vi "Vision_Right_PC_R3_RIO Test.vi"() -> ()   [LabVIEW 2015]
uses:
  <vilib>/vision/Pattern Matching.llb/IMAQ Curve Parameters.ctl
  <vilib>/vision/Pattern Matching.llb/IMAQ Match Range Setting.ctl
panel:
  in  "INITIAL Search Settings":T3={"Curve Parameters"={"Extraction Mode"=1, "Edge Threshold"=150, "Edge Filter Size"=0, "Min Length"=25, "Row Search Step Size"=15, "Col Search Step Size"=15, "Max Endpoint Gap"=2, "Closed"=TRUE, "Subpixel"=TRUE}, "Match Mode"={"Rotation"=TRUE, "Scale"=TRUE, "Occlusion"=FALSE, "Reserved"=FALSE, "Reserved"=FALSE, "Reserved"=FALSE}, "Range Settings"=[{"Match Constraints"=0, "Min"=-5.0, "Max"=5.0}, {"Match Constraints"=1, "Min"=50.0, "Max"=150.0}, {"Match Constraints"=2, "Min"=0.0, "Max"=0.0}], "Number of Matches"=1, "Minimum Match Score"=900.0, "SubPixel Accuracy"=TRUE, "Adv. Geometric Match Options 2"=[{"Setup Data Item"=20, "Item Value"=0.0}, {"Setup Data Item"=22, "Item Value"=1.0}]} {"Curve Parameters"."Extraction Mode" items=["Normal", "Uniform Regions"]; "Curve Parameters"."Edge Filter Size" items=["Fine", "Normal", "Contour Tracing"]; "Curve Parameters"."Max Endpoint Gap" min=0; "Curve Parameters"."Col Search Step Size" min=1 max=255 step=1; "Curve Parameters"."Row Search Step Size" min=1 max=255 step=1; "Curve Parameters"."Min Length" min=0; "Curve Parameters"."Edge Threshold" min=1 max=350 step=1; "Range Settings"."Max" format="%.2f"; "Range Settings"."Min" format="%.2f"; "Range Settings"."Match Constraints" items=["Rotation Angle (degrees)", "Scale Factor (%)", "Occlusion (%)"]; "Adv. Geometric Match Options 2"."Setup Data Item" items=["Curve Extraction Mode", "Curve Edge Threshold", "Curve Edge Filter Size", "Min Curve Length", "Curve Row Search Step Size", "Curve Col Search Step Size", "Curve Max Endpoint Gap", "Extract Closed Curves", "Enable Subpixel Curve Extraction", "Enable Correlation Score", "Enable Subpixel Accuracy", "Subpixel Iterations", "Subpixel Tolerance", "Initial Match List Length", "Enable Target Template Curve Score", "Min Match Separation Distance", "Min Match Separation Angle", "Min Match Separation Scale", "Max Match Overlap", "Enable Coarse Result", "Enable Calibration Support", "Enable Contrast Reversal", "Search Strategy", "Refinement Match Factor", "Subpixel Match Factor"]}
  in  "Timeout\nfail count":u16=100
  in  "Absolute\nMinimum Scale":dbl=10.0
  in  "Absolute\nMaximum Scale":dbl=300.0
  in  "Absolute\nMinimum Score":dbl=700.0
  in  "ROI_factor(vertical) LR":sgl=3.0
  in  "ROI_factor(Horiztonal) LR":sgl=6.0
  in  "LR to ST\nTransition Scale":sgl=150.0
  in  "SR to LR\nTransition Scale":sgl=70.0
  in  "Score\nCushion":dbl=50.0
  in  "Scale \nCushion":dbl=5.0
  in  "Default SR\nSetting Valuess":T4={"Min Scale"=20.0, "Max Scale"=200.0, "Min Score"=800.0}
  in  "Default LR\nSetting Values":T4={"Min Scale"=50.0, "Max Scale"=200.0, "Min Score"=800.0}
  in  "Default No Lock\nSetting Values":T4={"Min Scale"=20.0, "Max Scale"=250.0, "Min Score"=900.0}
  in  "Main ROI Decay\nper Fail (pixels)":i32=10
  in  "Indivudual Beacon \nCushion (pixels)":sgl=5.0
  out "Valid Scale History":dbl[](array[numeric])=[0.0, 0.0, 60.00346374511719, 0.0, 0.0, 0.0, 0.0, 0.0, 0.0, 0.0, 0.0, 0.0, 0.0, 0.0, 0.0, 0.0, 0.0, 0.0, 0.0, 0.0]
  out "Valid Score History":dbl[](array[numeric])=[0.0, 0.0, 905.1918334960938, 0.0, 0.0, 0.0, 0.0, 0.0, 0.0, 0.0, 0.0, 0.0, 0.0, 0.0, 0.0, 0.0, 0.0, 0.0, 0.0, 0.0]
  out "Valid Match History":bool[](array[boolean])=[FALSE, FALSE, TRUE, FALSE, FALSE, FALSE, FALSE, FALSE, FALSE, FALSE, FALSE, FALSE, FALSE, FALSE, FALSE, FALSE, FALSE, FALSE, FALSE, FALSE]
  out "Current State":u8
  out "Start Up":bool=TRUE
  out "New high Scale":dbl=250.0
  out "New Low Scale":dbl=20.0
  out "New Min Score":dbl=900.0
  out "Current Settings":T3={"Curve Parameters"={"Extraction Mode"=1, "Edge Threshold"=150, "Edge Filter Size"=0, "Min Length"=40, "Row Search Step Size"=15, "Col Search Step Size"=15, "Max Endpoint Gap"=2, "Closed"=TRUE, "Subpixel"=TRUE}, "Match Mode"={"Rotation"=TRUE, "Scale"=TRUE, "Occlusion"=FALSE, "Reserved"=FALSE, "Reserved"=FALSE, "Reserved"=FALSE}, "Range Settings"=[{"Match Constraints"=0, "Min"=-5.0, "Max"=5.0}, {"Match Constraints"=1, "Min"=20.0, "Max"=250.0}, {"Match Constraints"=2, "Min"=0.0, "Max"=0.0}], "Number of Matches"=1, "Minimum Match Score"=900.0, "SubPixel Accuracy"=TRUE, "Adv. Geometric Match Options 2"=[{"Setup Data Item"=20, "Item Value"=0.0}, {"Setup Data Item"=22, "Item Value"=1.0}]} {"Curve Parameters"."Extraction Mode" items=["Normal", "Uniform Regions"]; "Curve Parameters"."Edge Filter Size" items=["Fine", "Normal", "Contour Tracing"]; "Curve Parameters"."Max Endpoint Gap" min=0; "Curve Parameters"."Col Search Step Size" min=1 max=255 step=1; "Curve Parameters"."Row Search Step Size" min=1 max=255 step=1; "Curve Parameters"."Min Length" min=0; "Curve Parameters"."Edge Threshold" min=1 max=350 step=1; "Range Settings"."Max" format="%.2f"; "Range Settings"."Min" format="%.2f"; "Range Settings"."Match Constraints" items=["Rotation Angle (degrees)", "Scale Factor (%)", "Occlusion (%)"]}
  out "Current Score":sgl
  out "Current Scale":sgl
  out "Avg Scale":dbl=100.0
  out "Avg Score":dbl=750.0
  out "next ROI Rectangle 2":cluster{dbl, dbl, dbl, dbl, dbl}={87.0, 139.0, 527.0, 319.0, 0.0}
  in  "ROI_factor(vertical) SR":sgl=1.2
  in  "ROI_factor(Horiztonal) SR":sgl=6.0
  in  "Valid Treshold\nfor Lock":i16=5
  in  "History Size":i32=20
  out "Lock Status":bool
  out "SR Found":bool
  out "LR Found":bool
  out "Beacon 4 Data":cluster{"X":sgl, "Y":sgl}
  out "Beacon 3 Data":cluster{"X":sgl, "Y":sgl}={"X"=404.75333, "Y"=236.50656}
  out "Beacon 2 Data":cluster{"X":sgl, "Y":sgl}={"X"=305.31543, "Y"=230.27802}
  out "Beacon 1 Data":cluster{"X":sgl, "Y":sgl}={"X"=212.05559, "Y"=225.89603}
  out "Beacon 0 Data":cluster{"X":sgl, "Y":sgl}={"X"=128.98677, "Y"=232.05302}
  out "dT":u32=499
  out "Left Beacon Bools":bool[](array[boolean])
  out "Y Values":sgl[](array[numeric])=[232.05302, 225.89603, 230.27802, 236.50656, 0.0]
  out "X Values":sgl[](array[numeric])=[128.98677, 212.05559, 305.31543, 404.75333, 0.0]
  # "CURRENT VALUES"
  # "ADAPTIVE SETTINGS"
  # "Range"
  # "Range"
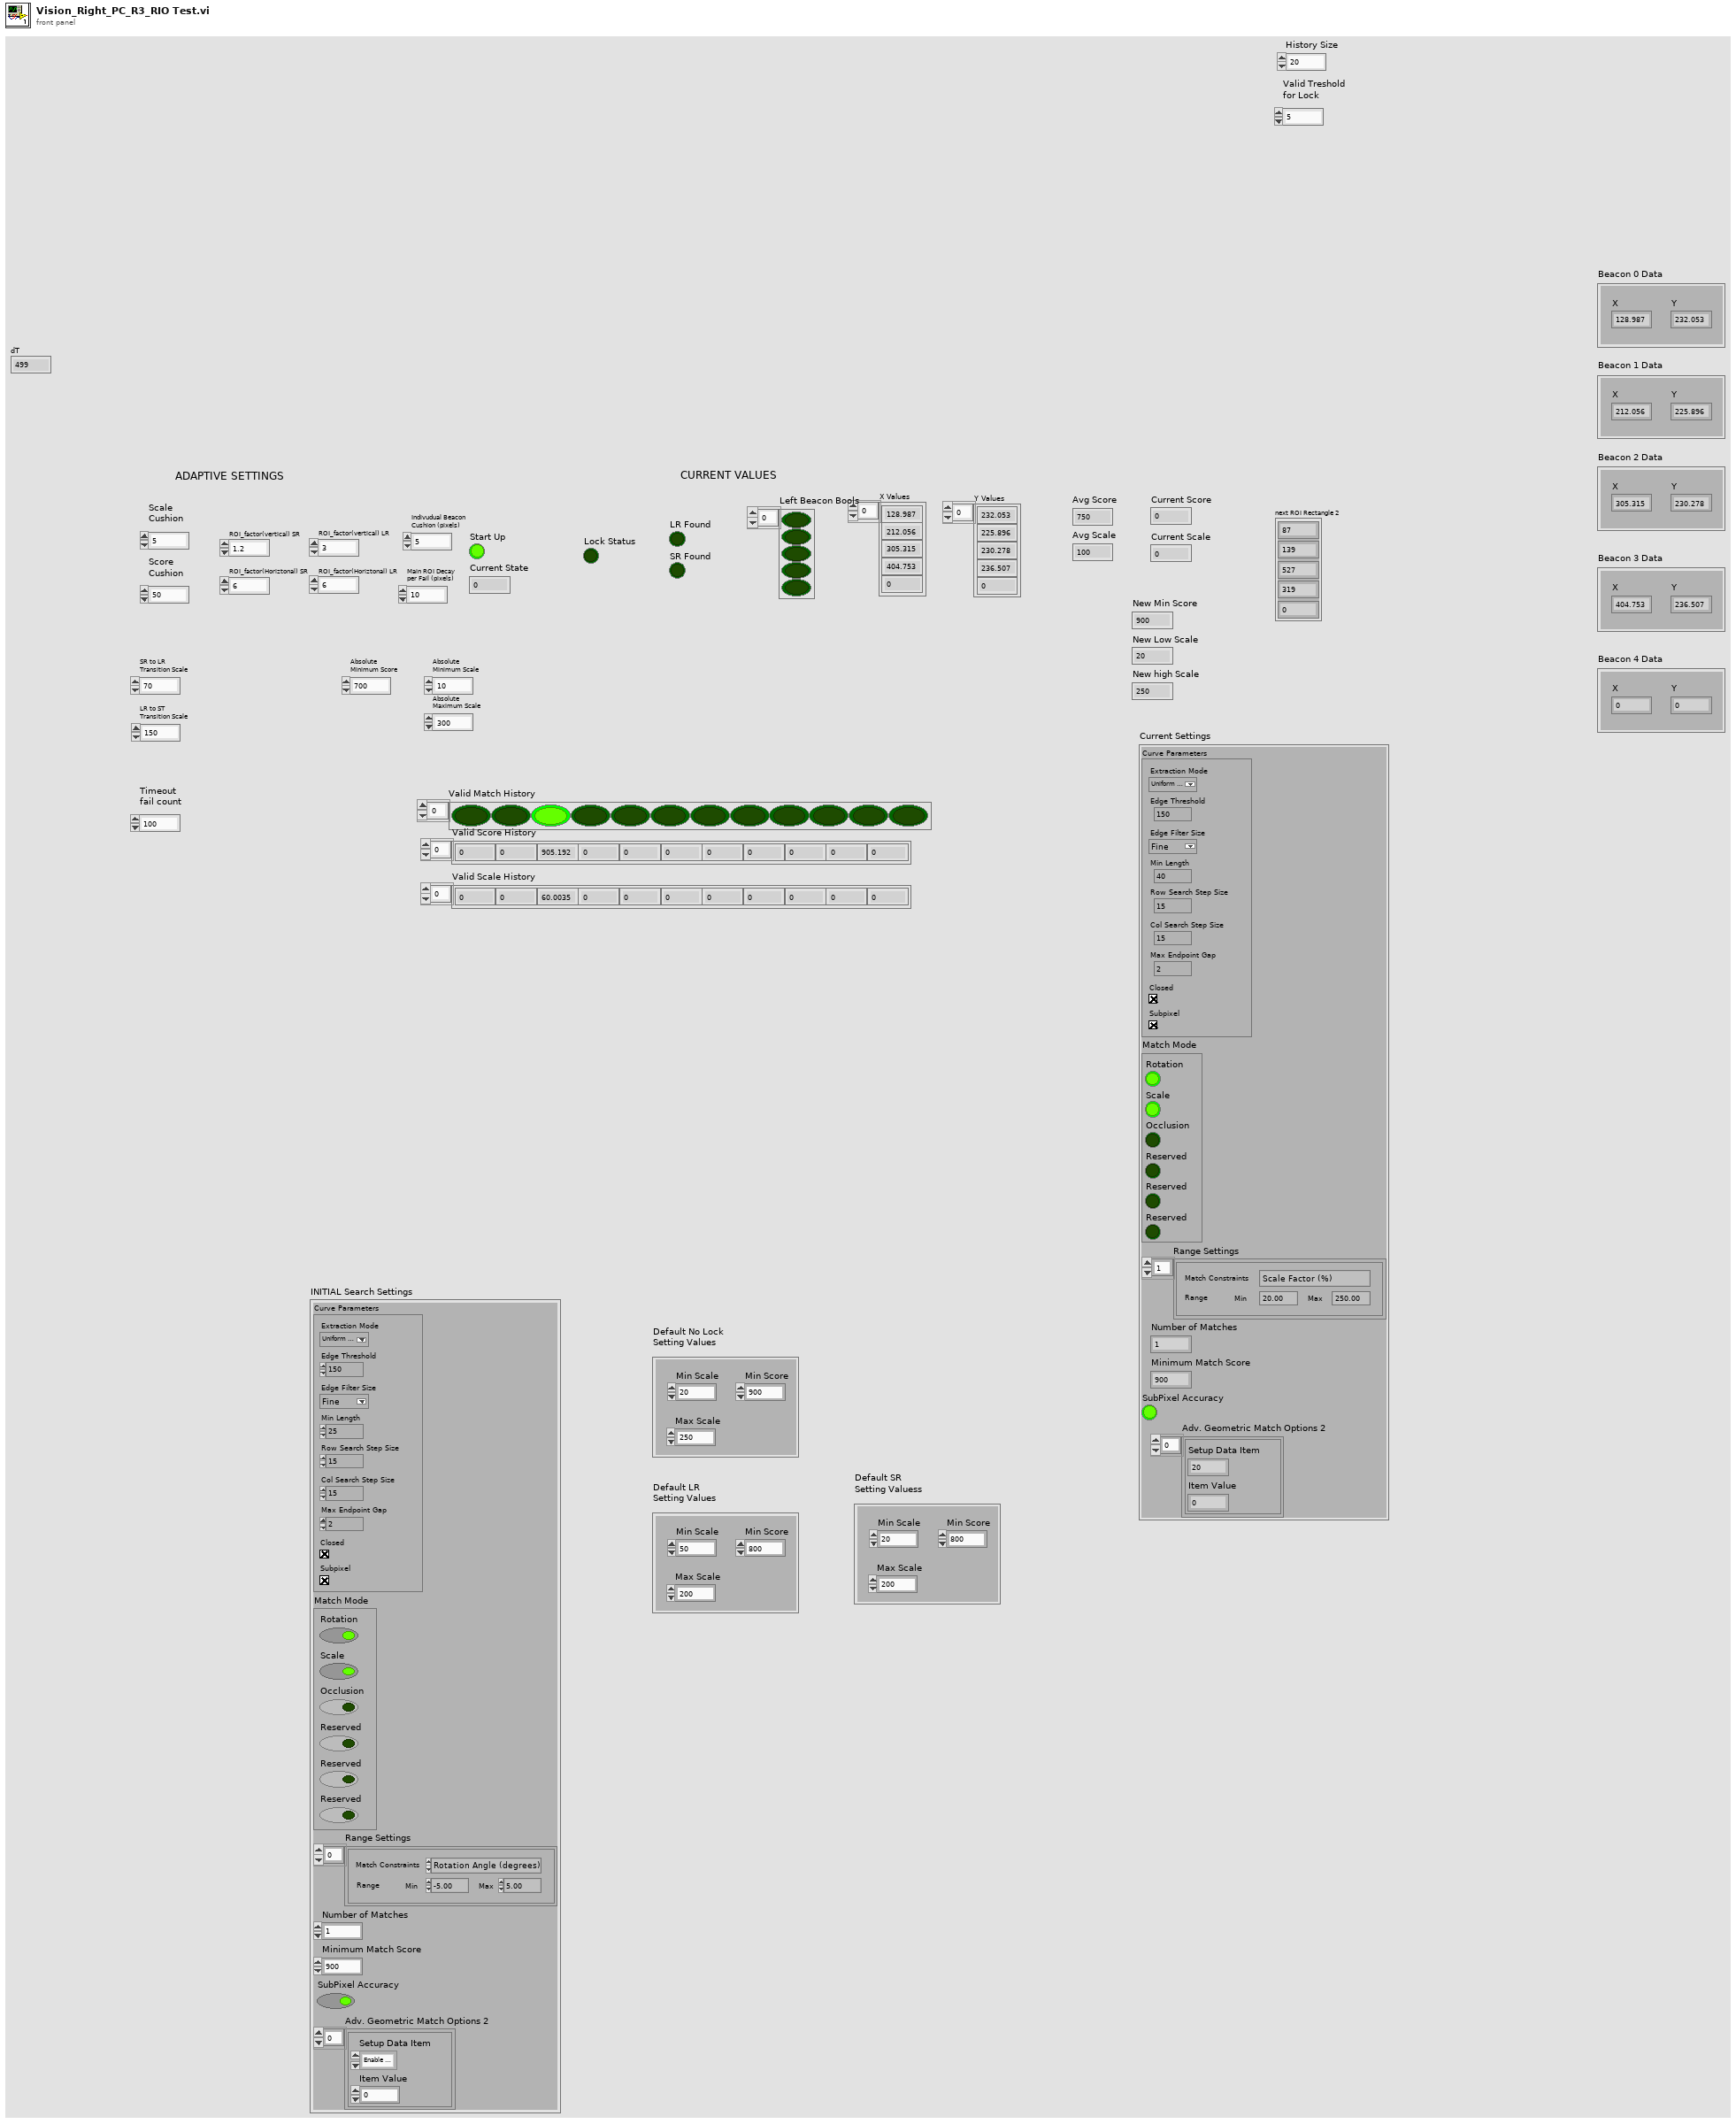
[diagram p1: front panel]
types:
  T1 = typedef "IMAQ Curve Parameters.ctl" = cluster{"Extraction Mode":u32, "Edge Threshold":i32, "Edge Filter Size":u32, "Min Length":i32, "Row Search Step Size":i32, "Col Search Step Size":i32, "Max Endpoint Gap":i32, "Closed":bool, "Subpixel":bool}
  T2 = typedef "IMAQ Match Range Setting.ctl" = cluster{"Match Constraints":u32, "Min":dbl, "Max":dbl}
  T3 = cluster{"Curve Parameters":T1, "Match Mode":cluster{"Rotation":bool, "Scale":bool, "Occlusion":bool, "Reserved":bool, "Reserved":bool, "Reserved":bool}, "Range Settings":T2[], "Number of Matches":i32, "Minimum Match Score":sgl, "SubPixel Accuracy":bool, "Adv. Geometric Match Options 2":cluster{"Setup Data Item":u16, "Item Value":dbl}[]}
  T4 = cluster{"Min Scale":dbl, "Max Scale":dbl, "Min Score":dbl}
  T5 = typedef "Image Type" = u32
  T6 = typedef "ROI Descriptor" = cluster{"Global Rectangle":i32[], "Contours":cluster{"ID":enum32{"External", "Internal"}, "Type":u32, "Coordinates":i32[]}[]}
  T7 = typedef "IMAQ Image.ctl" = refnum<image>
  T8 = typedef "IMAQ GM Match Report.ctl" = cluster{"Position":cluster{"x":sgl, "y":sgl}, "Angle":sgl, "Scale":sgl, "Score":sgl, "Bounding Box":cluster{"x":sgl, "y":sgl}[], "Contrast Reversed":bool, "Occlusion %":sgl, "Template Target Curve Score":sgl, "Target Template Curve Score":sgl, "Correlation Score":sgl}
  T9 = cluster{"Matches (Geometric Matching 1)[0]":T8, "Matches (Geometric Matching 1)[1]":T8, "Matches (Geometric Matching 1)[2]":T8, "Matches (Geometric Matching 1)[3]":T8, "Matches (Geometric Matching 1)[4]":T8, "Matches (Geometric Matching 1)[5]":T8, "Matches (Geometric Matching 1)[6]":T8, "Matches (Geometric Matching 1)[7]":T8, "Matches (Geometric Matching 1)[8]":T8}
  T10 = cluster{"Bounding Box[0]":cluster{"x":sgl, "y":sgl}, "Bounding Box[1]":cluster{"x":sgl, "y":sgl}, "Bounding Box[2]":cluster{"x":sgl, "y":sgl}, "Bounding Box[3]":cluster{"x":sgl, "y":sgl}, "Bounding Box[4]":cluster{"x":sgl, "y":sgl}, "Bounding Box[5]":cluster{"x":sgl, "y":sgl}, "Bounding Box[6]":cluster{"x":sgl, "y":sgl}, "Bounding Box[7]":cluster{"x":sgl, "y":sgl}, "Bounding Box[8]":cluster{"x":sgl, "y":sgl}}
  T11 = typedef "IMAQ Rectangle" = cluster{"Left":i32, "Top":i32, "Right":i32, "Bottom":i32, "Rotation":dbl}
  T12 = cluster{"index":u32, "Min Scale":dbl, "Max Scale":dbl}
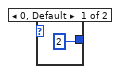
[diagram p2: hidden frame]
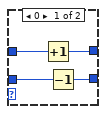
[diagram p4: hidden frame]
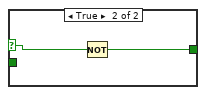
[diagram p5: hidden frame]
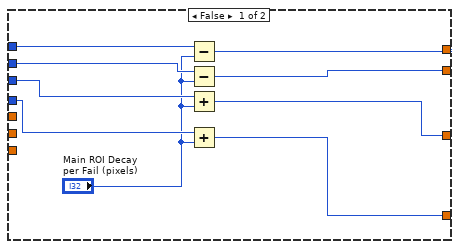
[diagram p6: hidden frame]
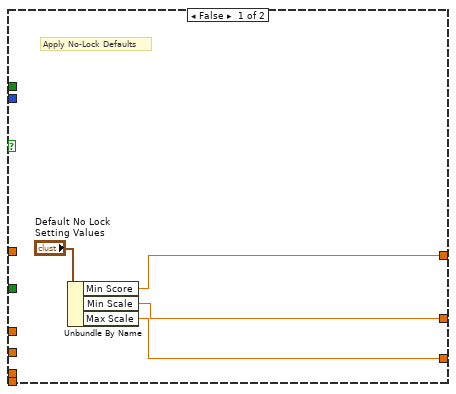
[diagram p11: hidden frame]
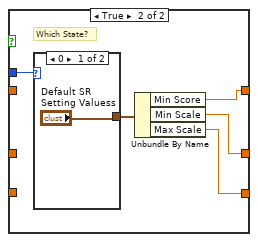
[diagram p12: hidden frame]
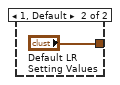
[diagram p13: hidden frame]
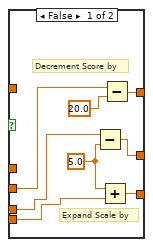
[diagram p14: hidden frame]
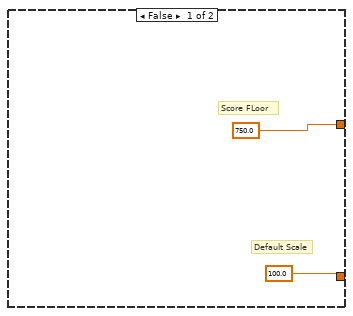
[diagram p15: hidden frame]
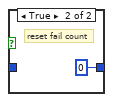
[diagram p17: hidden frame]
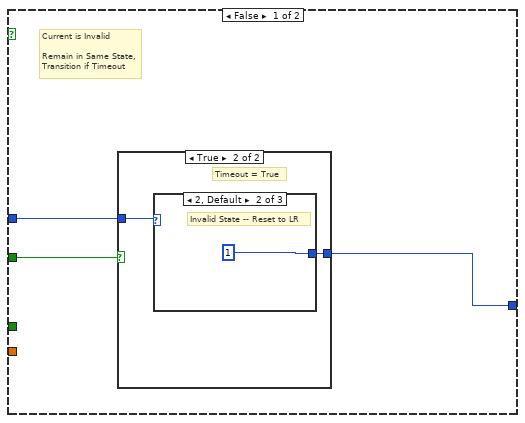
[diagram p18: hidden frame]
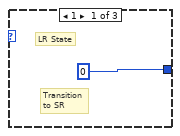
[diagram p20: hidden frame]
diagram:
  # "0 = Close Range (3)\n1 = Regular (5)"
  n1 = flat-sequence {
    tunnel: [w32] -> w12
    tunnel: [w29] -> w11
    tunnel: [w28] -> w10
    tunnel: ["INITIAL Search Settings"] -> w9
    tunnel: [u8 0] -> w8
    tunnel: [w24] -> w7
    tunnel: [FALSE] -> w6
    tunnel: [TRUE] -> w5
    tunnel: [w20] -> w4
    tunnel: [u16 0] -> w3
    tunnel: [w15] -> w2
    tunnel: [w14] -> w1
    tunnel: w12 -> [w46]
    tunnel: w11 -> [w51]
    tunnel: w10 -> [w49]
    tunnel: w9 -> [w47]
    tunnel: w8 -> [w50]
    tunnel: w7 -> [w48]
    tunnel: w6 -> [w45]
    tunnel: w5 -> [w44]
    tunnel: w4 -> [w43]
    tunnel: w3 -> [w42]
    tunnel: w2 -> [w41]
    tunnel: w1 -> [w40]
    frame #0 {
      w31 = T5 0 items=["Grayscale (U8)", "Grayscale (I16)", "Grayscale (SGL)", "Complex (CSG)", "RGB (U32)", "HSL (U32)", "RGB (U64)", "Grayscale (U16)"] ("Image Type")
      # "Score History"
      # "Scale History"
      # "Fail Counter"
      # "Valid Match History\n(main beacon)"
      # "Lock Status"
      # "Sub Beacon Search Array"
      # "Template State"
      # "Search Parameters"
      # "StartUp = True"
      # "Initial ROI Descriptor"
      # "INITIALIZE"
      n2 = Bundle(0, 0, 640, 480, 0) -> (w33:cluster{i32, i32, i32, i32, i32})  [unwired: 1 in]
      n3 = call "IMAQ Convert Rectangle to ROI"("Rectangle"=w33) -> ("ROI Descriptor"=w32:T6)  [unwired: 8 in, 1 out]
      n4 = Initialize Array(FALSE, 5 ("dimension size")) -> (w24:bool[])
      n5 = Initialize Array(FALSE, "History Size") -> (w20:bool[])
      n6 = Initialize Array(0.0, "History Size") -> (w14:dbl[])
      n7 = Initialize Array(0.0, "History Size") -> (w15:dbl[])
      n8 = call "IMAQ Create"("Image Name"="Right_Image", "Image Type"=w31) -> ("New Image"=w28:T7, "error out"=w29:errorcluster)  [unwired: 3 in]
    }
    frame #1 {
      # "Fail Counter"
      # "Template State"
      # "Score History"
      # "Scale History"
      # "Valid Match History\n(main beacon)"
      # "Lock Status"
      # "Sub Beacon Search Array"
      # "StartUp"
      n9 = call "Tick Count3"() -> ("Tick Count(uSec)"=w39:u32)
      n10 = while {
        tunnel: w51 -> [w84]
        shift-right: [w76] -> _
        shift-left: w50 -> [w80]
        shift-right: [w68] -> _
        shift-left: w44 -> [w69]
        tunnel: w49 -> [w81]
        shift-right: [w67] -> _
        shift-left: w48 -> [w79]
        shift-right: [w72] -> _
        shift-left: w47 -> [w73]
        shift-right: [w70] -> _
        shift-left: w46 -> [w71]
        shift-right: [w66] -> _
        shift-left: w45 -> [_]
        shift-right: [w63] -> _
        shift-left: w43 -> [w78]
        shift-right: [w62] -> _
        shift-left: w42 -> [w77]
        shift-right: [w64] -> _
        shift-left: w41 -> [w75]
        shift-right: [w65] -> _
        shift-left: w40 -> [w74]
        shift-right: [w59] -> _
        shift-left: w39 -> [w60]
        stop <- FALSE stop-if-true
        n11 = flat-sequence {
          tunnel: w84 -> [w88]
          tunnel: [w87] -> w83
          tunnel: [w86] -> w82
          tunnel: [w85] -> w52
          tunnel: w83 -> [w271]
          tunnel: w82 -> [w270]
          tunnel: w81 -> [w254]
          tunnel: w69 -> [w269]
          tunnel: w80 -> [w127]
          tunnel: w79 -> [w268]
          tunnel: w73 -> [w126]
          tunnel: w71 -> [w267]
          tunnel: w78 -> [w208]
          tunnel: w73 -> [w188]
          tunnel: w77 -> [w204]
          tunnel: [w114] -> w76
          tunnel: w75 -> [w139]
          tunnel: w74 -> [w140]
          tunnel: [w186] -> w72
          tunnel: w71 -> [w159]
          tunnel: w69 -> [w152]
          tunnel: [w149] -> w65
          tunnel: [w148] -> w64
          tunnel: [w147] -> w63
          tunnel: [w146] -> w62
          tunnel: w60 -> [w142]
          tunnel: [w157] -> w58
          tunnel: [w156] -> w57
          tunnel: [w151] -> w56
          tunnel: [w150] -> w55
          tunnel: [w118] -> w54
          tunnel: [w141] -> w53
          tunnel: w52 -> [w91]
          tunnel: [w701] -> w59
          tunnel: [w702] -> w66
          tunnel: [w703] -> w67
          tunnel: [w704] -> w68
          tunnel: [w705] -> _
          tunnel: [w706] -> w70
          tunnel: w58 -> [w706]
          tunnel: w57 -> [w705]
          tunnel: w56 -> [w704]
          tunnel: w55 -> [w703]
          tunnel: w54 -> [w702]
          tunnel: w53 -> [w701]
          frame #0 {
            # "Take Image"
            n12 = shared-variable "RT myRIO Target - Overlord\\Localization_Variables_r0.lvlib\\Right Servo Angle_Current"() -> (w85:dbl)  [unwired: 1 in, 1 out]
            n13 = call "Right Camera Acquisition"("error in"=w88) -> ("Image Out"=w86:T7, "error out"=w87:errorcluster)  [unwired: 24 in, 1 out]
          }
          frame #1 {
            w89 = sgl 240.0 ("y")
            w90 = sgl 320.0 ("y")
            w189 = u32 1 ("index")
            (unwired) 0
            # "Apply Limits to Settings"
            # "Choose ROI Scale Factor"
            # "Current Min\n& Max Scale"
            # "fail count out"
            # "Next State"
            # "Have fail count threshold to reset to worst case scenario settings, have treshold less than timeout"
            # "False case*********"
            # "Make new templates for sub beacons based on \noriginal template... import pic to express VI\n\n\nUse scale window for smaller beacons"
            # "Outer Beacon\nIndexes"
            # "Build ROI for Individual Beacons Based on Main Bounding Box"
            # "Maybe check for main here"
            # "Startup FLag"
            # "Pull Down Startup IF Already True and Lock\nOtherwise don't update"
            # "ROI"
            # "State Change"
            # "Next Settings"
            # "Settings out"
            # "Scale"
            # "Min Score"
            # "Lower Scale"
            # "Upper Scale"
            # "If Locked"
            # "Average Scale"
            # "Average Score"
            # "Only Calculate\nAvg if 2 available"
            # "Valid  Ccount\n(up to 3)"
            # "Only Calculate MOving Avg\nif xx% of previous positions were valid"
            # "Update Avg Score & Scale"
            # "Timeout"
            # "Update Fail Counter"
            # "Next State"
            # "Settings"
            # "Update Template State"
            # "Update Main ROI"
            # "Update Search Setting Values"
            # "Current Match is Valid \nIF: \n     Main Found\n     At Least 2 or 3 beacons"
            # "****# of previous in history that must be true\nin order for position to be considered \"locked\""
            # "Shift & Insert Current Valid Match"
            # "Update Lock Status & Shift Arrays"
            # "Main Found"
            # "Update Beacon Outputs"
            # "Valid Match"
            # "Valid Match"
            # "Valid Match"
            # "Valid Match"
            # "Assume 0 Angle"
            # "Starting X Lower Bound"
            # "Length of\nIndividual Beacon ROI"
            # "Length of Bounding Box"
            # "LR Found"
            # "SR Found"
            # "Valid Match"
            # "Only Attempt Sub If Supposed To"
            # "Search for Sub Beacons"
            # "Force SR if Start Up"
            # "Choose Template (SR or LR)\n& Search"
            n14 = case shown="True" w269 {
              tunnel: w127 -> [w635 _]
              tunnel: [w635 u8 1] -> w95
              frame False {
                # "Not Start Up\n\nDon't Update \nTemplate State"
              }
              frame True {
                # "Start Up --> SR"
              }
            }
            "Current State" <- w95
            n15 = shared-variable "RT myRIO Target - Overlord\\Localization_Variables_r0.lvlib\\Right Servo Angle_Image"(w91) -> ()  [unwired: 1 in, 1 out]
            n16 = case shown="1" w95 {
              tunnel: w271 -> [w651 w683]
              tunnel: w270 -> [w650 w682]
              tunnel: w254 -> [w649 w681]
              tunnel: w268 -> [w646 w677]
              tunnel: w126 -> [w645 w671]
              tunnel: w267 -> [w644 w670]
              tunnel: [w643 w676] -> w150
              tunnel: [sgl 3.0 ("y") sgl 5.0 ("y")] -> w253
              tunnel: [w641 w673] -> w155
              tunnel: [w640 w672] -> w158
              tunnel: [w639 FALSE] -> w216
              tunnel: [FALSE w675] -> w217
              frame 0, Default {
                # "Sub-Beacon Search\nArray"
                n17 = call "Left Camera - Short Range"("Image In"=w650, "Image Dst"=w649, "ROI Descriptor (Geometric Matching 1)"=w644, "Settings (Geometric Matching 1)"=w645, "Template File Path (Geometric Matching 1)"=path "/home/lvuser/natinst/bin/BeaconTemplates_TEST/Close Range (3 subs).png", "error in"=w651) -> ("Image Out"=w641:T7, "Matches (Geometric Matching 1)"=w640:T8[], "Number of Matches (Geometric Matching 1)"=w648:i32)  [unwired: 18 in, 1 out]
                n18 = Equal?(x=w648, y=1) -> (x = y?=w639:bool)
                n19 = case shown="True" w639 {
                  tunnel: w646 -> [w659 w663]
                  tunnel: [w652 w660] -> w643
                  frame False {
                    w653 = FALSE
                    # "No Main Found,\nDon't Search any Subs"
                    n20 = Replace Array Subset(array=w659, new element #1=w653, index #1=0 ("y"), new element #2=w653, index #2=1 ("y"), new element #3=w653, index #3=2 ("y"), new element #4=w653, index #4=3 ("y"), new element #5=w653, index #5=4 ("y")) -> (w652:bool[])
                  }
                  frame True {
                    w661 = TRUE
                    w662 = FALSE
                    # "Search for Middle 3 Subs"
                    n21 = Replace Array Subset(array=w663, new element #1=w662, index #1=0 ("y"), new element #2=w661, index #2=1 ("y"), new element #3=w661, index #3=2 ("y"), new element #4=w661, index #4=3 ("y"), new element #5=w662, index #5=4 ("y")) -> (w660:bool[])
                  }
                }
              }
              frame 1 {
                # "Main (5) Pattern"
                n22 = call "Left Camera - Long Range"("Image In"=w682, "Image Dst"=w681, "ROI Descriptor (Geometric Matching 1)"=w670, "Settings (Geometric Matching 1)"=w671, "Template File Path (Geometric Matching 1)"=path "/home/lvuser/natinst/bin/BeaconTemplates_TEST/Main Beacon_8ft - 320_240.png", "error in"=w683) -> ("Image Out"=w673:T7, "Matches (Geometric Matching 1)"=w672:T8[], "Number of Matches (Geometric Matching 1)"=w678:i32)  [unwired: 18 in, 1 out]
                n23 = Equal?(x=w678, y=1) -> (x = y?=w675:bool)
                n24 = case shown="True" w675 {
                  tunnel: w677 -> [w691 w693]
                  tunnel: [w684 w692] -> w676
                  frame False {
                    w685 = FALSE
                    # "F"
                    # "No Main Found,\nDon't Search any Subs"
                    n25 = Replace Array Subset(array=w691, new element #1=w685, index #1=0 ("y"), new element #2=w685, index #2=1 ("y"), new element #3=w685, index #3=2 ("y"), new element #4=w685, index #4=3 ("y"), new element #5=w685, index #5=4 ("y")) -> (w684:bool[])
                  }
                  frame True {
                    w694 = TRUE
                    # "T"
                    # "Search for ALL Beacons"
                    n26 = Replace Array Subset(array=w693, new element #1=w694, index #1=0 ("y"), new element #2=w694, index #2=1 ("y"), new element #3=w694, index #3=2 ("y"), new element #4=w694, index #4=3 ("y"), new element #5=w694, index #5=4 ("y")) -> (w692:bool[])
                  }
                }
              }
            }
            "LR Found" <- w217
            "SR Found" <- w216
            n27 = Array To Cluster(array=w158) -> (cluster=w138:T9)
            n28 = Unbundle By Name(w138) -> ("Matches (Geometric Matching 1)[0].Bounding Box"=w255:cluster{"x":sgl, "y":sgl}[], "Matches (Geometric Matching 1)[0].Scale"=w195:sgl, "Matches (Geometric Matching 1)[0].Correlation Score"=w154:sgl)
            "Current Scale" <- w195
            "Current Score" <- w154
            n29 = Or(x=w217, y=w216) -> (x .or. y?=w209:bool)
            n30 = Array To Cluster(array=w255) -> (cluster=w266:T10)
            n31 = Unbundle By Name(w266) -> ("Bounding Box[0].x"=w250:sgl, "Bounding Box[0].y"=w137:sgl, "Bounding Box[2].x"=w248:sgl, "Bounding Box[2].y"=w135:sgl)
            n32 = Subtract(x=w248, y=w250) -> (x-y=w252:sgl)
            n33 = case shown="1, Default" w95 {
              tunnel: [w279 w283] -> w130
              tunnel: [w278 w282] -> w129
              tunnel: 0 -> [w281 w283]
              tunnel: 4 -> [w280 w282]
              frame 0 {
                n34 = Increment(x=w281) -> (x+1=w279:i32)
                n35 = Decrement(x=w280) -> (x-1=w278:i32)
              }
              frame 1, Default {
              }
            }
            n36 = Divide(x=w252, y=w253) -> (x/y=w249:sgl)
            n37 = Subtract(x=w137, y="Indivudual Beacon \nCushion (pixels)") -> (x-y=w136:sgl)
            n38 = Add(x="Indivudual Beacon \nCushion (pixels)", y=w135) -> (x+y=w134:sgl)
            n39 = for {
              N: 5 -> [_]
              tunnel: w150 -> [w496] mode=indexing
              shift-right: [w480] -> _
              shift-left: w250 -> [w495]
              tunnel: w249 -> [w494]
              tunnel: w136 -> [w493]
              tunnel: w134 -> [w492]
              tunnel: [w489] -> w131 mode=indexing
              tunnel: w130 -> [w486]
              tunnel: w129 -> [w487]
              tunnel: "Indivudual Beacon \nCushion (pixels)" -> [w477]
              i -> [w488]
              # "Apply Horizontal Cushion to Outer Beacons"
              # "Divide Bounding Box"
              # "Upper Bound of Current is\nLower Bound for Next"
              # "Build ROI\nDescriptor"
              n40 = case shown="True" w496 {
                tunnel: w495 -> [w509 w510]
                tunnel: w494 -> [_ w512]
                tunnel: [w509 w511] -> w478
                tunnel: [w509 w510] -> w483
                frame False {
                  # "Don't Care"
                }
                frame True {
                  # "X Lower Bound"
                  n41 = Add(x=w510, y=w512) -> (x+y=w511:sgl)
                }
              }
              n42 = Equal?(x=w488, y=w486) -> (x = y?=w485:bool)
              n43 = case shown="True" w485 {
                tunnel: w483 -> [w504 w508]
                tunnel: [w504 w505] -> w482
                tunnel: [w503 w506] -> w479
                tunnel: w478 -> [w503 w506]
                tunnel: w477 -> [_ w507]
                frame False {
                }
                frame True {
                  n44 = Subtract(x=w508, y=w507) -> (x-y=w505:sgl)
                }
              }
              n45 = Equal?(x=w488, y=w487) -> (x = y?=w484:bool)
              n46 = case shown="True" w484 {
                tunnel: w482 -> [w498 w502]
                tunnel: [w498 w501] -> w481
                tunnel: [w497 w499] -> w480
                tunnel: w479 -> [w497 w499]
                tunnel: w477 -> [_ w500]
                frame False {
                }
                frame True {
                  n47 = Add(x=w502, y=w500) -> (x+y=w501:sgl)
                }
              }
              n48 = Bundle("x"=w481, w493, "x"=w480, w492, 0) -> (w490:cluster{"x":sgl, sgl, "x":sgl, sgl, i32})  [unwired: 1 in]
              n49 = call "IMAQ Convert Rectangle to ROI"("Rectangle"=w490) -> ("ROI Descriptor"=w489:T6)  [unwired: 8 in, 1 out]
            }
            n50 = Index Array(array=w150, index=1) -> (element=w259:bool)
            n51 = Index Array(array=w131, index=1) -> (element=w241:T6)
            n52 = Index Array(array=w150, index=2) -> (element=w258:bool)
            n53 = Index Array(array=w131, index=2) -> (element=w240:T6)
            n54 = Index Array(array=w150, index=0) -> (element=w265:bool)
            n55 = Index Array(array=w131, index=3) -> (element=w239:T6)
            n56 = Index Array(array=w150, index=3) -> (element=w257:bool)
            n57 = Index Array(array=w131, index=4) -> (element=w238:T6)
            n58 = Index Array(array=w131, index=0) -> (element=w242:T6)
            n59 = Index Array(array=w150, index=4) -> (element=w256:bool)
            n60 = case shown="True" w259 {
              tunnel: w241 -> [_ w601]
              tunnel: w155 -> [_ w600]
              tunnel: w254 -> [_ w599]
              tunnel: [FALSE w592] -> w236
              tunnel: w95 -> [_ w591]
              tunnel: w126 -> [_ w590]
              frame False {
              }
              frame True {
                # "Update Beacon Coordinates if Found"
                n61 = case shown="1, Default" w591 {
                  tunnel: w601 -> [w606 w615]
                  tunnel: w600 -> [w608 w614]
                  tunnel: w599 -> [w607 w613]
                  tunnel: [w604 w612] -> w594
                  tunnel: [w605 w611] -> w593
                  tunnel: w590 -> [w603 w610]
                  frame 0 {
                    n62 = call "Mid Left Match Short Range"("Image In"=w608, "Image Dst"=w607, "ROI Descriptor (Geometric Matching 1)"=w606, "Settings (Geometric Matching 1)"=w603, "Template File Path (Geometric Matching 1)"=path "/home/lvuser/natinst/bin/BeaconTemplates_TEST/sub2_SR.png") -> ("Matches (Geometric Matching 1)"=w605:T8[], "Number of Matches (Geometric Matching 1)"=w604:i32)  [unwired: 19 in, 2 out]
                  }
                  frame 1, Default {
                    n63 = call "Mid Left Match Long Range"("Image In"=w614, "Image Dst"=w613, "ROI Descriptor (Geometric Matching 1)"=w615, "Settings (Geometric Matching 1)"=w610, "Template File Path (Geometric Matching 1)"=path "/home/lvuser/natinst/bin/BeaconTemplates_TEST/sub2_8ft - 320_240.png") -> ("Matches (Geometric Matching 1)"=w611:T8[], "Number of Matches (Geometric Matching 1)"=w612:i32)  [unwired: 19 in, 2 out]
                  }
                }
                n64 = Array To Cluster(array=w593) -> (cluster=w598:T9)
                n65 = Equal?(x=w594, y=1) -> (x = y?=w592:bool)
                n66 = Unbundle By Name(w598) -> ("Matches (Geometric Matching 1)[0].Position.x"=w596:sgl, "Matches (Geometric Matching 1)[0].Position.y"=w595:sgl)
                n67 = case shown="True" w592 {
                  tunnel: w596 -> [_ w618]
                  tunnel: w595 -> [_ w617]
                  frame False {
                  }
                  frame True {
                    n68 = Bundle("x"=w618, "y"=w617) -> (→"Beacon 1 Data":cluster{"x":sgl, "y":sgl})  [unwired: 1 in]
                  }
                }
              }
            }
            n69 = case shown="True" w258 {
              tunnel: w240 -> [_ w562]
              tunnel: w155 -> [_ w571]
              tunnel: w254 -> [_ w570]
              tunnel: [FALSE w563] -> w235
              tunnel: w95 -> [_ w561]
              tunnel: w126 -> [_ w560]
              frame False {
              }
              frame True {
                # "Update Beacon Coordinates if Found"
                n70 = case shown="1, Default" w561 {
                  tunnel: w571 -> [w578 w585]
                  tunnel: w570 -> [w577 w584]
                  tunnel: [w575 w583] -> w565
                  tunnel: [w574 w582] -> w564
                  tunnel: w562 -> [w576 w581]
                  tunnel: w560 -> [w573 w580]
                  frame 0 {
                    n71 = call "Middle Match Short Range"("Image In"=w578, "Image Dst"=w577, "ROI Descriptor (Geometric Matching 1)"=w576, "Settings (Geometric Matching 1)"=w573, "Template File Path (Geometric Matching 1)"=path "/home/lvuser/natinst/bin/BeaconTemplates_TEST/sub3_SR.png") -> ("Matches (Geometric Matching 1)"=w575:T8[], "Number of Matches (Geometric Matching 1)"=w574:i32)  [unwired: 19 in, 2 out]
                  }
                  frame 1, Default {
                    n72 = call "Middle Match Long Range"("Image In"=w585, "Image Dst"=w584, "ROI Descriptor (Geometric Matching 1)"=w581, "Settings (Geometric Matching 1)"=w580, "Template File Path (Geometric Matching 1)"=path "/home/lvuser/natinst/bin/BeaconTemplates_TEST/sub3_8ft - 320_240.png") -> ("Matches (Geometric Matching 1)"=w583:T8[], "Number of Matches (Geometric Matching 1)"=w582:i32)  [unwired: 19 in, 2 out]
                  }
                }
                n73 = Array To Cluster(array=w565) -> (cluster=w569:T9)
                n74 = Equal?(x=w564, y=1) -> (x = y?=w563:bool)
                n75 = Unbundle By Name(w569) -> ("Matches (Geometric Matching 1)[0].Position.x"=w567:sgl, "Matches (Geometric Matching 1)[0].Position.y"=w566:sgl)
                n76 = case shown="True" w563 {
                  tunnel: w567 -> [_ w588]
                  tunnel: w566 -> [_ w587]
                  frame False {
                  }
                  frame True {
                    n77 = Bundle("x"=w588, "y"=w587) -> (→"Beacon 2 Data":cluster{"x":sgl, "y":sgl})  [unwired: 1 in]
                  }
                }
              }
            }
            n78 = case shown="True" w257 {
              tunnel: w239 -> [_ w541]
              tunnel: w155 -> [_ w540]
              tunnel: w254 -> [_ w539]
              tunnel: [FALSE w532] -> w234
              tunnel: w95 -> [_ w531]
              tunnel: w126 -> [_ w530]
              frame False {
              }
              frame True {
                # "Update Beacon Coordinates if Found"
                n79 = case shown="1, Default" w531 {
                  tunnel: w541 -> [w546 w555]
                  tunnel: w540 -> [w548 w554]
                  tunnel: w539 -> [w547 w553]
                  tunnel: [w545 w552] -> w534
                  tunnel: [w544 w551] -> w533
                  tunnel: w530 -> [w543 w550]
                  frame 0 {
                    n80 = call "Mid Right Match Short Range"("Image In"=w548, "Image Dst"=w547, "ROI Descriptor (Geometric Matching 1)"=w546, "Settings (Geometric Matching 1)"=w543, "Template File Path (Geometric Matching 1)"=path "/home/lvuser/natinst/bin/BeaconTemplates_TEST/sub4_SR.png") -> ("Matches (Geometric Matching 1)"=w544:T8[], "Number of Matches (Geometric Matching 1)"=w545:i32)  [unwired: 19 in, 2 out]
                  }
                  frame 1, Default {
                    n81 = call "Mid Right Match Long Range"("Image In"=w554, "Image Dst"=w553, "ROI Descriptor (Geometric Matching 1)"=w555, "Settings (Geometric Matching 1)"=w550, "Template File Path (Geometric Matching 1)"=path "/home/lvuser/natinst/bin/BeaconTemplates_TEST/sub4_8ft - 320_240.png") -> ("Matches (Geometric Matching 1)"=w551:T8[], "Number of Matches (Geometric Matching 1)"=w552:i32)  [unwired: 19 in, 2 out]
                  }
                }
                n82 = Array To Cluster(array=w533) -> (cluster=w538:T9)
                n83 = Equal?(x=w534, y=1) -> (x = y?=w532:bool)
                n84 = Unbundle By Name(w538) -> ("Matches (Geometric Matching 1)[0].Position.x"=w536:sgl, "Matches (Geometric Matching 1)[0].Position.y"=w535:sgl)
                n85 = case shown="True" w532 {
                  tunnel: w536 -> [_ w558]
                  tunnel: w535 -> [_ w557]
                  frame False {
                  }
                  frame True {
                    n86 = Bundle("x"=w558, "y"=w557) -> (→"Beacon 3 Data":cluster{"x":sgl, "y":sgl})  [unwired: 1 in]
                  }
                }
              }
            }
            n87 = case shown="True" w265 {
              tunnel: w242 -> [_ w627]
              tunnel: w155 -> [_ w626]
              tunnel: w254 -> [_ w625]
              tunnel: [FALSE w622] -> w237
              tunnel: w126 -> [_ w621]
              frame False {
              }
              frame True {
                # "Update Beacon Coordinates if Found"
                n88 = call "Far Left Match2"("Image In"=w626, "Image Dst"=w625, "ROI Descriptor (Geometric Matching 1)"=w627, "Settings (Geometric Matching 1)"=w621, "Template File Path (Geometric Matching 1)"=path "/home/lvuser/natinst/bin/BeaconTemplates_TEST/sub1_8ft - 320_240.png") -> ("Matches (Geometric Matching 1)"=w629:T8[], "Number of Matches (Geometric Matching 1)"=w628:i32)  [unwired: 19 in, 2 out]
                n89 = Array To Cluster(array=w629) -> (cluster=w631:T9)
                n90 = Equal?(x=w628, y=1) -> (x = y?=w622:bool)
                n91 = Unbundle By Name(w631) -> ("Matches (Geometric Matching 1)[0].Position.x"=w624:sgl, "Matches (Geometric Matching 1)[0].Position.y"=w623:sgl)
                n92 = case shown="True" w622 {
                  tunnel: w624 -> [_ w634]
                  tunnel: w623 -> [_ w633]
                  frame False {
                  }
                  frame True {
                    n93 = Bundle("x"=w634, "y"=w633) -> (→"Beacon 0 Data":cluster{"x":sgl, "y":sgl})  [unwired: 1 in]
                  }
                }
              }
            }
            n94 = case shown="True" w256 {
              tunnel: w238 -> [_ w525]
              tunnel: w155 -> [_ w524]
              tunnel: w254 -> [_ w523]
              tunnel: [FALSE w516] -> w233
              tunnel: w126 -> [_ w515]
              frame False {
              }
              frame True {
                # "Update Beacon Coordinates if Found"
                n95 = call "Far Right Match Long Range"("Image In"=w524, "Image Dst"=w523, "ROI Descriptor (Geometric Matching 1)"=w525, "Settings (Geometric Matching 1)"=w515, "Template File Path (Geometric Matching 1)"=path "/home/lvuser/natinst/bin/BeaconTemplates_TEST/sub5_8ft - 320_240.png") -> ("Matches (Geometric Matching 1)"=w518:T8[], "Number of Matches (Geometric Matching 1)"=w517:i32)  [unwired: 19 in, 2 out]
                n96 = Array To Cluster(array=w518) -> (cluster=w522:T9)
                n97 = Equal?(x=w517, y=1) -> (x = y?=w516:bool)
                n98 = Unbundle By Name(w522) -> ("Matches (Geometric Matching 1)[0].Position.x"=w520:sgl, "Matches (Geometric Matching 1)[0].Position.y"=w519:sgl)
                n99 = case shown="True" w516 {
                  tunnel: w520 -> [_ w528]
                  tunnel: w519 -> [_ w527]
                  frame False {
                  }
                  frame True {
                    n100 = Bundle("x"=w528, "y"=w527) -> (→"Beacon 4 Data":cluster{"x":sgl, "y":sgl})  [unwired: 1 in]
                  }
                }
              }
            }
            n101 = local read "Beacon 0 Data"() -> (w232:cluster{"X":sgl, "Y":sgl})
            n102 = local read "Beacon 1 Data"() -> (w231:cluster{"X":sgl, "Y":sgl})
            n103 = local read "Beacon 2 Data"() -> (w230:cluster{"X":sgl, "Y":sgl})
            n104 = local read "Beacon 3 Data"() -> (w229:cluster{"X":sgl, "Y":sgl})
            n105 = local read "Beacon 4 Data"() -> (w228:cluster{"X":sgl, "Y":sgl})
            n106 = Build Array(w237, w236, w235, w234, w233) -> (w94:bool[])
            "Left Beacon Bools" <- w94
            n107 = Unbundle(w232) -> ("X"=w227:sgl, "Y"=w222:sgl)
            n108 = Unbundle(w231) -> ("X"=w226:sgl, "Y"=w221:sgl)
            n109 = Unbundle(w230) -> ("X"=w225:sgl, "Y"=w220:sgl)
            n110 = Unbundle(w228) -> ("X"=w223:sgl, "Y"=w218:sgl)
            n111 = Unbundle(w229) -> ("X"=w224:sgl, "Y"=w219:sgl)
            n112 = shared-variable "RT myRIO Target - Overlord\\Localization_Variables_r0.lvlib\\RIGHT_BEACON_BOOL_array"(w94) -> ()  [unwired: 1 in, 1 out]
            n113 = Build Array(w227, w226, w225, w224, w223) -> (w93:sgl[])
            "X Values" <- w93
            n114 = Build Array(w222, w221, w220, w219, w218) -> (w92:sgl[])
            "Y Values" <- w92
            n115 = shared-variable "RT myRIO Target - Overlord\\Localization_Variables_r0.lvlib\\RIGHT_BEACON_Y_array"(w92) -> ()  [unwired: 1 in, 1 out]
            n116 = shared-variable "RT myRIO Target - Overlord\\Localization_Variables_r0.lvlib\\RIGHT_BEACON_X_array"(w93) -> ()  [unwired: 1 in, 1 out]
            n117 = Boolean To (0,1)(Boolean=w94) -> (0, 1=w213:i16[])
            n118 = case shown="1" w95 {
              tunnel: [2 i16 2 ("y")] -> w211
              frame 0, Default {
              }
              frame 1 {
              }
            }
            n119 = Add Array Elements(numeric array=w213) -> (sum=w212:i16)
            n120 = Greater Or Equal?(x=w212, y=w211) -> (x >= y?=w210:bool)
            n121 = And(x=w209, y=w210) -> (x .and. y?=w119:bool)
            n122 = case shown="False" w119 {
              tunnel: w204 -> [w402 _]
              tunnel: [w401 u16 0] -> w146
              frame False {
                n123 = Increment(x=w402) -> (x+1=w401:u16)
              }
              frame True {
                # "reset fail count"
              }
            }
            n124 = local read "History Size"() -> (w207:i32)
            n125 = Decrement(x=w207) -> (x-1=w206:i32)
            n126 = for {
              N: w207 -> [_]
              shift-right: [w455] -> w147
              shift-left: w208 -> [w454]
              tunnel: w119 -> [w453]
              tunnel: w206 -> [w449]
              shift-right: [w446] -> w149
              shift-left: w140 -> [w448]
              shift-right: [w445] -> w148
              shift-left: w139 -> [w447]
              tunnel: w195 -> [w444]
              tunnel: w154 -> [w443]
              i -> [w452]
              # "Reverse Index"
              n127 = Subtract(x=w449, y=w452) -> (x-y=w450:i32)
              n128 = Equal To 0?(x=w450) -> (x = 0?=w451:bool)
              n129 = case shown="True" w451 {
                tunnel: w450 -> [w456 w473]
                tunnel: w454 -> [w466 w475]
                tunnel: [w464 w476] -> w455
                tunnel: w453 -> [_ w474]
                tunnel: w448 -> [w461 w472]
                tunnel: w447 -> [w460 w471]
                tunnel: [w459 w467] -> w446
                tunnel: [w458 w468] -> w445
                tunnel: w444 -> [_ w470]
                tunnel: w443 -> [_ w469]
                frame False {
                  # "Shift Old"
                  n130 = Decrement(x=w456) -> (x-1=w457:i32)
                  n131 = Index Array(array=w466, index=w457) -> (element=w465:bool)
                  n132 = Index Array(array=w461, index=w457) -> (element=w463:dbl)
                  n133 = Index Array(array=w460, index=w457) -> (element=w462:dbl)
                  n134 = Replace Array Subset(array=w466, new element=w465, index=w456) -> (w464:bool[])
                  n135 = Replace Array Subset(array=w461, new element=w463, index=w456) -> (w459:dbl[])
                  n136 = Replace Array Subset(array=w460, new element=w462, index=w456) -> (w458:dbl[])
                }
                frame True {
                  # "Scale"
                  # "Score"
                  # "Valid"
                  # "insert New"
                  n137 = Replace Array Subset(array=w472, new element=w469, index=w473) -> (w467:dbl[])
                  n138 = Replace Array Subset(array=w471, new element=w470, index=w473) -> (w468:dbl[])
                  n139 = Replace Array Subset(array=w475, new element=w474, index=w473) -> (w476:bool[])
                }
              }
            }
            "Valid Match History" <- w147
            "Valid Score History" <- w149
            "Valid Scale History" <- w148
            n140 = Initialize Array(u8 0, u8 3) -> (w200:u8[])
            n141 = local read "History Size"() -> (w199:i32)
            n142 = while {
              shift-right: [w383] -> w201
              shift-left: w200 -> [w385]
              tunnel: w147 -> [w392] mode=indexing
              shift-right: [w390] -> w193
              shift-left: u8 0 -> [w393]
              tunnel: w199 -> [w391]
              i -> [w384]
              stop <- w386 stop-if-true
              # "Grab Last 2 Valid Indexes"
              n143 = case shown="True" w392 {
                tunnel: w393 -> [w395 w397]
                tunnel: [w395 w400] -> w390
                tunnel: w385 -> [w394 w399]
                tunnel: w384 -> [_ w398]
                tunnel: [w394 w396] -> w383
                frame False {
                }
                frame True {
                  # "Update Index\nto use"
                  # "Increment\nValid Count"
                  n144 = Replace Array Subset(array=w399, new element=w398, index=w397) -> (w396:u8[])
                  n145 = Increment(x=w397) -> (x+1=w400:u8)
                }
              }
              n146 = Greater?(x=w384, y=w391) -> (0:w387:bool)
              n147 = Greater Or Equal?(x=w390, y=u8 3) -> (x >= y?=w388:bool)
              n148 = Or(x=w388, y=w387) -> (x .or. y?=w386:bool)
            }
            n149 = Boolean To (0,1)(Boolean=w147) -> (0, 1=w215:i16[])
            n150 = Add Array Elements(numeric array=w215) -> (sum=w214:i16)
            n151 = Greater Or Equal?(x=w214, y="Valid Treshold\nfor Lock") -> (x >= y?=w118:bool)
            "Lock Status" <- w118
            n152 = Equal?(x=w193, y=u8 3) -> (x = y?=w194:bool)
            n153 = case shown="True" w194 {
              tunnel: w201 -> [_ w379]
              tunnel: w149 -> [_ w378]
              tunnel: [750.0 w372] -> w191
              tunnel: w148 -> [_ w363]
              tunnel: [100.0 w362] -> w185
              frame False {
                # "Default Scale"
                # "Score FLoor"
              }
              frame True {
                # "Average"
                # "Average"
                # "Grab Last 2 Valid Score Values"
                n154 = Index Array(array=w379, index=u8 0) -> (element=w366:u8)
                n155 = Index Array(array=w379, index=u8 1) -> (element=w365:u8)
                n156 = Index Array(array=w379, index=u8 2) -> (element=w364:u8)
                n157 = Index Array(array=w378, index=w366) -> (element=w377:dbl)
                n158 = Index Array(array=w378, index=w365) -> (element=w376:dbl)
                n159 = Index Array(array=w378, index=w364) -> (element=w375:dbl)
                n160 = Index Array(array=w363, index=w366) -> (element=w371:dbl)
                n161 = Index Array(array=w363, index=w365) -> (element=w370:dbl)
                n162 = Index Array(array=w363, index=w364) -> (element=w369:dbl)
                n163 = Compound Arithmetic op=ADD(w377, w376, w375) -> (w374:dbl)
                n164 = Compound Arithmetic op=ADD(w371, w370, w369) -> (w368:dbl)
                n165 = Divide(x=w374, y=3.0) -> (x/y=w372:dbl)
                n166 = Divide(x=w368, y=3.0) -> (x/y=w362:dbl)
              }
            }
            "Avg Score" <- w191
            "Avg Scale" <- w185
            n167 = call "Tick Count2"() -> ("Tick Count(uSec)"=w141:u32)
            n168 = Subtract(x=w141, y=w142) -> (x-y=w145:u32)
            n169 = Divide(x=w145, y=u32 1000) -> (x/y=→"dT":dbl)
            n170 = Array To Cluster(array=w158) -> (cluster=w175:T9)
            n171 = Unbundle By Name(w175) -> ("Matches (Geometric Matching 1)[0].Position.x"=w166:sgl, "Matches (Geometric Matching 1)[0].Position.y"=w165:sgl, "Matches (Geometric Matching 1)[0].Scale"=w164:sgl)
            n172 = call "IMAQ Convert ROI to Rectangle"("ROI Descriptor"=w159) -> ("Rectangle"=w184:T11)  [unwired: 8 in, 1 out]
            n173 = Greater Or Equal?(x=w146, y="Timeout\nfail count") -> (x >= y?=w202:bool)
            n174 = Unbundle By Name(w184) -> ("Left"=w170:i32, "Top"=w169:i32, "Right"=w168:i32, "Bottom"=w167:i32)
            n175 = case shown="True" w119 {
              tunnel: w185 -> [_ w419]
              tunnel: w118 -> [_ w418]
              tunnel: w95 -> [w405 w417]
              tunnel: [w404 w416] -> w114
              tunnel: w202 -> [w406 w415]
              tunnel: "SR to LR\nTransition Scale" -> [_ w414]
              tunnel: "LR to ST\nTransition Scale" -> [_ w413]
              frame False {
                # "Current is Invalid\n\nRemain in Same State,\nTransition if Timeout"
                n176 = case shown="True" w406 {
                  tunnel: w405 -> [w407 w409]
                  tunnel: [w407 w408] -> w404
                  frame False {
                    # "Retain Current State until Timeout"
                  }
                  frame True {
                    # "Timeout = True"
                    n177 = case shown="2, Default" w409 {
                      tunnel: [u8 0 u8 1 u8 1] -> w408
                      frame 1 {
                        # "Transition\nto SR"
                        # "LR State"
                      }
                      frame 2, Default {
                        # "Invalid State -- Reset to LR"
                      }
                      frame 0 {
                        # "Transition\nto LR"
                        # "SR State"
                      }
                    }
                  }
                }
              }
              frame True {
                # "Timeout"
                # "Lock Status"
                # "Only update if Current is Valid"
                # "Scale"
                # "Current State"
                n178 = case shown="1" w417 {
                  selector: w417 -> [w422 _ w434]
                  tunnel: w419 -> [w427 _ w440]
                  tunnel: w418 -> [w425 _ w439]
                  tunnel: [w421 u8 1 w435] -> w416
                  tunnel: w415 -> [w423 _ w433]
                  tunnel: w414 -> [_ _ w432]
                  tunnel: w413 -> [w420 _ _]
                  frame 1 {
                    # "Switch to LR if \ntimeout\nor Scale & Lock"
                    # "% Scale to transition to SR"
                    # "LR State"
                    n179 = Greater Or Equal?(x=w427, y=w420) -> (x >= y?=w424:bool)
                    n180 = And(x=w425, y=w424) -> (x .and. y?=w426:bool)
                    n181 = Or(x=w423, y=w426) -> (x .or. y?=w428:bool)
                    n182 = case shown="True" w428 {
                      tunnel: [w429 u8 0] -> w421
                      tunnel: w422 -> [w429 _]
                      frame False {
                        # "Retain Current\nState"
                      }
                      frame True {
                        # "Transition\nto SR"
                      }
                    }
                  }
                  frame 2, Default {
                    # "Invalid State -- Reset to LR"
                  }
                  frame 0 {
                    # "Switch to LR if \ntimeout\nor Scale & Lock"
                    # "SR State"
                    # "% Scale to transition to LR"
                    n183 = Less Or Equal?(x=w440, y=w432) -> (x <= y?=w438:bool)
                    n184 = And(x=w439, y=w438) -> (x .and. y?=w436:bool)
                    n185 = Or(x=w433, y=w436) -> (x .or. y?=w437:bool)
                    n186 = case shown="False" w437 {
                      tunnel: [w441 u8 1] -> w435
                      tunnel: w434 -> [w441 _]
                      frame False {
                        # "Retain Current\nState"
                      }
                      frame True {
                      }
                    }
                  }
                }
              }
            }
            n187 = case shown="1" w114 {
              tunnel: "ROI_factor(vertical) SR" -> [w275 _]
              tunnel: "ROI_factor(Horiztonal) SR" -> [w274 _]
              tunnel: "ROI_factor(vertical) LR" -> [_ w277]
              tunnel: "ROI_factor(Horiztonal) LR" -> [_ w276]
              tunnel: [w275 w277] -> w109
              tunnel: [w274 w276] -> w108
              frame 0, Default {
              }
              frame 1 {
              }
            }
            n188 = case shown="True" w119 {
              tunnel: w164 -> [_ w298]
              tunnel: w166 -> [_ w305]
              tunnel: w165 -> [_ w300]
              tunnel: [w290 w306] -> w160
              tunnel: [w289 w299] -> w163
              tunnel: [w288 w304] -> w162
              tunnel: [w287 w302] -> w161
              tunnel: w170 -> [w295 _]
              tunnel: w169 -> [w294 _]
              tunnel: w168 -> [w293 _]
              tunnel: w167 -> [w292 _]
              tunnel: w109 -> [_ w297]
              tunnel: w108 -> [_ w296]
              frame False {
                n189 = Subtract(x=w295, y="Main ROI Decay\nper Fail (pixels)") -> (x-y=w290:i32)
                n190 = Subtract(x=w294, y="Main ROI Decay\nper Fail (pixels)") -> (x-y=w289:i32)
                n191 = Add(x=w293, y="Main ROI Decay\nper Fail (pixels)") -> (x+y=w288:i32)
                n192 = Add(x=w292, y="Main ROI Decay\nper Fail (pixels)") -> (x+y=w287:i32)
              }
              frame True {
                # "Horizontal Scale \n(smaller number = smaller ROI)"
                # "Vertical Scale \n(larger number = smaller ROI)"
                # "If continuous beacon found then adjust ROI appropriately."
                n193 = Divide(x=w298, y=w297) -> (x/y=w303:sgl)
                n194 = Multiply(x=w298, y=w296) -> (x*y=w308:sgl)
                n195 = Divide(x=w308, y=sgl 2.0) -> (x/y=w301:sgl)
                n196 = Add(x=w300, y=w303) -> (x+y=w302:sgl)
                n197 = Subtract(x=w300, y=w303) -> (x-y=w299:sgl)
                n198 = Subtract(x=w305, y=w301) -> (x-y=w306:sgl)
                n199 = Add(x=w305, y=w301) -> (x+y=w304:sgl)
              }
            }
            n200 = Less?(x=w160, y=sgl 0.0) -> (x < y?=w181:bool)
            n201 = Less?(x=w163, y=sgl 0.0) -> (x < y?=w180:bool)
            n202 = Greater?(x=w161, y=w89) -> (0:w177:bool)
            n203 = Greater?(x=w162, y=w90) -> (0:w179:bool)
            n204 = Unbundle By Name(w188) -> ("Minimum Match Score"=w120:sgl, "Range Settings"=w124:T2[])
            n205 = Not Equal?(x=w114, y=w95) -> (x != y?=w117:bool)
            n206 = case shown="True" w181 {
              tunnel: [w315 0.0] -> w171
              tunnel: w160 -> [w315 _]
              frame False {
              }
              frame True {
              }
            }
            n207 = case shown="True" w180 {
              tunnel: [w309 0.0] -> w172
              tunnel: w163 -> [w309 _]
              frame False {
              }
              frame True {
              }
            }
            n208 = case shown="True" w179 {
              tunnel: [w311 w312] -> w173
              tunnel: w162 -> [w311 _]
              tunnel: w90 -> [_ w312]
              frame False {
              }
              frame True {
              }
            }
            n209 = case shown="True" w177 {
              tunnel: [w313 w314] -> w174
              tunnel: w161 -> [w313 _]
              tunnel: w89 -> [_ w314]
              frame False {
              }
              frame True {
              }
            }
            n210 = Index Array(array=w124, index=u32 1) -> (element=w123:T2)
            n211 = Unbundle(w123) -> ("Min"=w122:dbl, "Max"=w121:dbl)  [unwired: 1 out]
            n212 = case shown="True" w118 {
              tunnel: w191 -> [_ w334]
              tunnel: w185 -> [_ w333]
              tunnel: [w319 w326] -> w105
              tunnel: [w318 w325] -> w101
              tunnel: [w317 w324] -> w97
              tunnel: w122 -> [_ w331]
              tunnel: w121 -> [_ w330]
              tunnel: w120 -> [_ w332]
              tunnel: w119 -> [_ w329]
              tunnel: w117 -> [_ w328]
              tunnel: w114 -> [_ w327]
              frame False {
                # "Apply No-Lock Defaults"
                n213 = Unbundle By Name("Default No Lock\nSetting Values") -> ("Min Score"=w319:dbl, "Min Scale"=w318:dbl, "Max Scale"=w317:dbl)
              }
              frame True {
                # "Apply Default Template State Settings\nIF Transitioning \nTemplate States"
                # "Check if Current is True"
                n214 = case shown="True" w329 {
                  tunnel: w334 -> [_ w359]
                  tunnel: [w347 w358] -> w323
                  tunnel: w333 -> [_ w357]
                  tunnel: [w346 w356] -> w322
                  tunnel: [w345 w355] -> w321
                  tunnel: w332 -> [w350 _]
                  tunnel: w331 -> [w349 _]
                  tunnel: w330 -> [w348 _]
                  frame False {
                    w351 = 5.0 ("y")
                    # "Expand Scale by"
                    # "Decrement Score by"
                    n215 = Subtract(x=w349, y=w351) -> (x-y=w346:dbl)
                    n216 = Add(x=w351, y=w348) -> (x+y=w345:dbl)
                    n217 = Subtract(x=w350, y=20.0) -> (x-y=w347:dbl)
                  }
                  frame True {
                    n218 = Subtract(x=w359, y="Score\nCushion") -> (x-y=w358:dbl)
                    n219 = Subtract(x=w357, y="Scale \nCushion") -> (x-y=w356:dbl)
                    n220 = Add(x="Scale \nCushion", y=w357) -> (x+y=w355:dbl)
                  }
                }
                n221 = case shown="False" w328 {
                  tunnel: w327 -> [_ w342]
                  tunnel: [w337 w340] -> w326
                  tunnel: [w336 w339] -> w325
                  tunnel: [w335 w338] -> w324
                  tunnel: w323 -> [w337 _]
                  tunnel: w322 -> [w336 _]
                  tunnel: w321 -> [w335 _]
                  frame False {
                    # "No State Change,\nkeep previous values"
                  }
                  frame True {
                    # "Which State?"
                    n222 = case shown="0" w342 {
                      tunnel: ["Default SR\nSetting Valuess" "Default LR\nSetting Values"] -> w341
                      frame 0 {
                      }
                      frame 1, Default {
                      }
                    }
                    n223 = Unbundle By Name(w341) -> ("Min Score"=w340:dbl, "Min Scale"=w339:dbl, "Max Scale"=w338:dbl)
                  }
                }
              }
            }
            n224 = Bundle(w171, w172, "y"=w173, "y"=w174, 0.0) -> (w176:cluster{dbl, dbl, "y":sgl, "y":sgl, dbl})  [unwired: 1 in]
            "next ROI Rectangle 2" <- w176
            n225 = call "IMAQ Convert Rectangle to ROI"("Rectangle"=w176) -> ("ROI Descriptor"=w157:T6)  [unwired: 8 in, 1 out]
            n226 = Bundle(w171, w172, "y"=w173, "y"=w174) -> (w156:cluster{dbl, dbl, "y":sgl, "y":sgl})  [unwired: 1 in]
            n227 = Less?(x=w105, y="Absolute\nMinimum Score") -> (x < y?=w107:bool)
            n228 = Less?(x=w101, y="Absolute\nMinimum Scale") -> (x < y?=w103:bool)
            n229 = Greater?(x=w97, y="Absolute\nMaximum Scale") -> (0:w99:bool)
            n230 = Select(t="Absolute\nMinimum Score", s=w107, f=w105) -> (s? t:f=w104:dbl)
            "New Min Score" <- w104
            n231 = Select(t="Absolute\nMinimum Scale", s=w103, f=w101) -> (s? t:f=w100:dbl)
            "New Low Scale" <- w100
            n232 = Select(t="Absolute\nMaximum Scale", s=w99, f=w97) -> (s? t:f=w96:dbl)
            "New high Scale" <- w96
            n233 = Bundle("index"=w189, "Min Scale"=w100, "Max Scale"=w96) -> (w190:T12)  [unwired: 1 in]
            n234 = Replace Array Subset(array=w124, new element=w190, index=w189) -> (w187:T2[])
            n235 = Bundle By Name(cluster=w188, "Range Settings"=w187, "Minimum Match Score"=w104) -> (w186:T3)
            n236 = And(x=w118, y=w152) -> (x .and. y?=w153:bool)
            n237 = case shown="False" w153 {
              selector: w153 -> [_ w286]
              tunnel: [w284 w285] -> w151
              tunnel: w152 -> [w284 _]
              frame False {
              }
              frame True {
                n238 = Not(x=w286) -> (.not. x?=w285:bool)
              }
            }
            "Current Settings" <- w126
          }
          frame #2 {
            n239 = shared-variable "RT myRIO Target - Overlord\\Localization_Variables_r0.lvlib\\RIGHT_FLAG"(TRUE ("Left_Flag")) -> ()  [unwired: 1 in, 1 out]
          }
        }
        "Start Up" <- w69
      }
    }
  }
